vi "Module Cleanup.vi"(8 "error in (no error)":errorcluster, 11 "System Status Module in":refnum<class "System Status Module.lvclass">) -> (0 "error out":errorcluster, 3 "System Status Module out":refnum<class "System Status Module.lvclass">)   [LabVIEW 2020, in "VolatusGUI.lvlib" / "System Status Module.lvclass"]
uses:
  System Status Module.lvclass
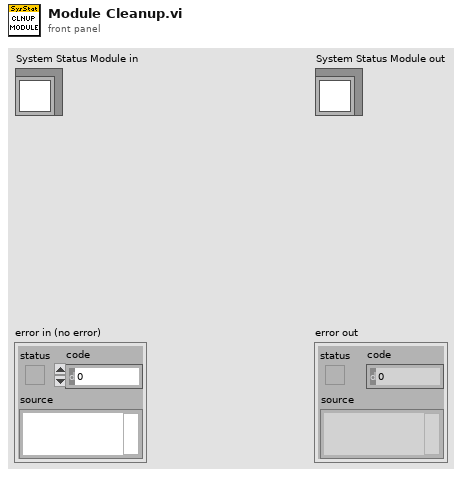
[diagram p1: front panel]
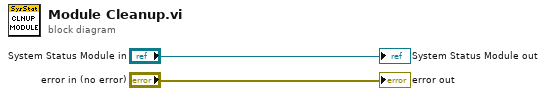
[diagram p0: block diagram]
diagram:
  "error out" <- "error in (no error)"
  "System Status Module out" <- "System Status Module in"
